vi "Round to Nearest Time Slot.vi"(8 "Error In":errorcluster, 10 "Time Slot Size (ms)":dbl, 11 "Duration (s)":dbl) -> (0 "Error Out":errorcluster, 2 "Slots Count":i32, 3 "Nearest Time Slot (s)":dbl)   [LabVIEW 2019, in "Motion Profile Generator.lvclass"]
uses:
  Motion Profile Generator.lvclass
  <vilib>/ErrorRing/Error Ring.xnode
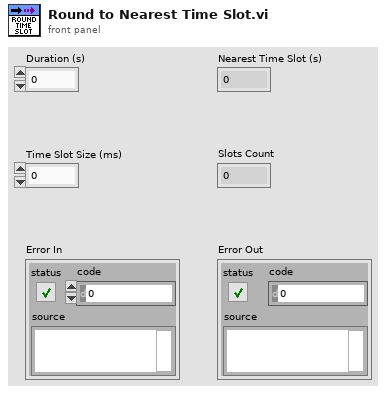
[diagram p1: front panel]
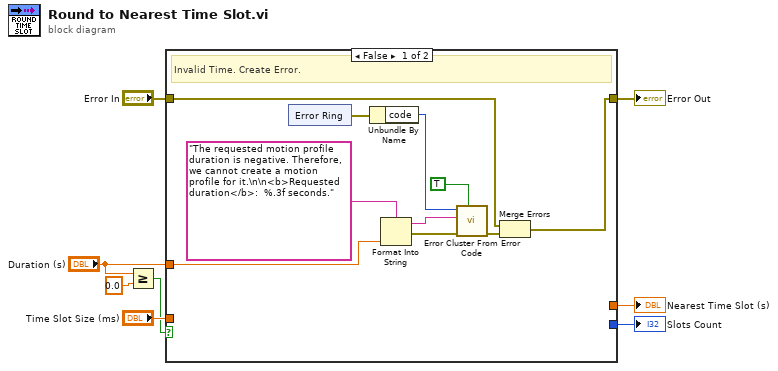
[diagram p0: block diagram]
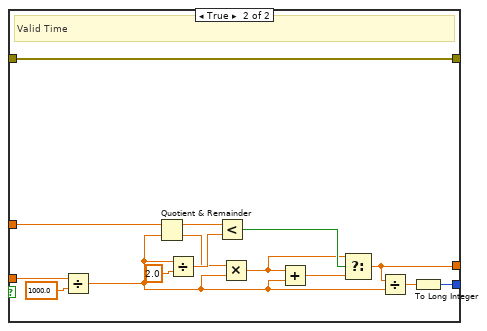
[diagram p2: hidden frame]
diagram:
  n1 = Greater Or Equal?(x="Duration (s)", y=0.0) -> (x >= y?=w3:bool)
  n2 = case shown="False" w3 {
    tunnel: [_ w30] -> w8
    tunnel: "Time Slot Size (ms)" -> [_ w29]
    tunnel: "Duration (s)" -> [w10 w26]
    tunnel: [_ w24] -> w4
    tunnel: "Error In" -> [w18 w23]
    tunnel: [w17 w23] -> w1
    frame False {
      # "Invalid Time. Create Error."
      n3 = xnode "Error Ring"() -> ("error out"=w14:errorcluster)
      n4 = Unbundle By Name(w14) -> ("code"=w13:i32)
      n5 = Format Into String(format string="The requested motion profile duration is negative. Therefore, we cannot create a motion profile for it.\n\n<b>Requested duration</b>:  %.3f seconds.", w10) -> (resulting string=w12:string, error out=w11:errorcluster)  [unwired: 2 in]
      n6 = call <vilib>:"Error Cluster From Error Code.vi"("show call chain? (False)"=TRUE, "error in (no error)"=w11, "error message (\"\")"=w12, "error code (0)"=w13) -> ("error out"=w16:errorcluster)  [unwired: 5 in]
      n7 = Merge Errors(w18, w16) -> (w17:errorcluster)
    }
    frame True {
      # "Valid Time"
      n8 = Divide(x=w29, y=1000.0 ("x")) -> (x/y=w28:dbl)
      n9 = Quotient & Remainder(x=w26, y=w28) -> (x-y*floor(x/y)=w34:dbl, floor(x/y)=w33:dbl)
      n10 = Divide(x=w28, y=2.0) -> (x/y=w36:dbl)
      n11 = Less?(x=w34, y=w36) -> (x < y?=w37:bool)
      n12 = Multiply(x=w33, y=w28) -> (x*y=w31:dbl)
      n13 = Add(x=w31, y=w28) -> (x+y=w32:dbl)
      n14 = Select(t=w31, s=w37, f=w32) -> (s? t:f=w30:dbl)
      n15 = Divide(x=w30, y=w28) -> (x/y=w25:dbl)
      n16 = To Long Integer(number=w25) -> (32bit integer=w24:i32)
    }
  }
  "Nearest Time Slot (s)" <- w8
  "Slots Count" <- w4
  "Error Out" <- w1
